vi "From Byte Array (U32).vi"(1 "byte array in":u8[](array[numeric]) format="%x") -> (0 "element out":u32)   [LabVIEW 2015, in "ni579x Config v2 Shared.lvlib"]
uses:
  <instrlib>/ni579x/Config/v2/Shared/ni579x Config v2 Shared.lvlib
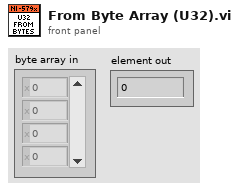
[diagram p1: front panel]
types:
  T1 = enum16{"big-endian, network order", "native, host order", "little-endian"}
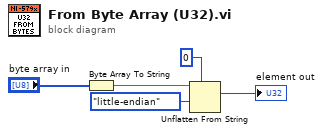
[diagram p0: block diagram]
diagram:
  n1 = Byte Array To String(unsigned byte array="byte array in") -> (string=w5:string)
  n2 = Unflatten From String(type=u32 0, binary string=w5, byte order (0:big-endian, network order)=T1."little-endian") -> (value=→"element out":u32)  [unwired: 2 in, 2 out]
